vi "Library.RemoveDuplicates.vi"(8 "error in (no error)":errorcluster, 11 "Library References":refnum<vi>[](array[refnum])) -> (0 "error out":errorcluster, 3 "Library References (no duplicates)":refnum<vi>[](array[refnum]))   [LabVIEW 2011]
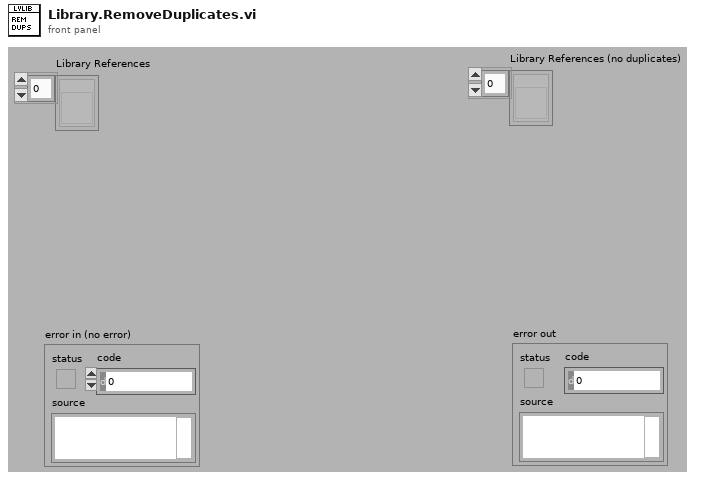
[diagram p1: front panel]
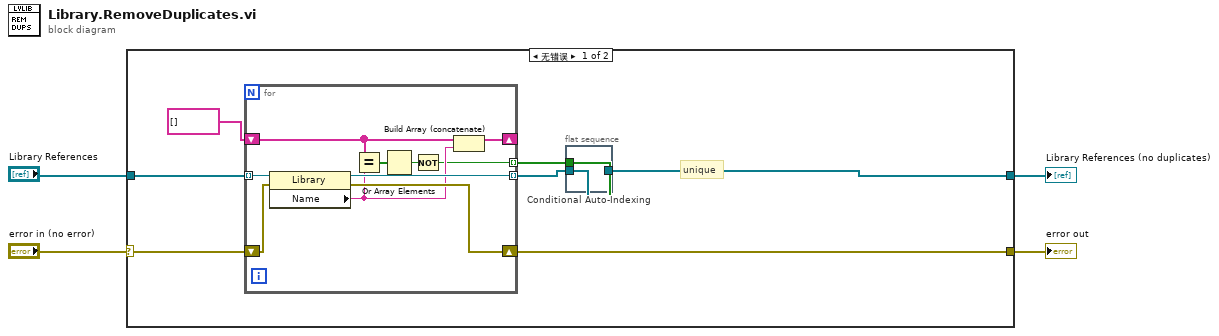
[diagram p0: block diagram]
diagram:
  n1 = case shown="无错误" "error in (no error)" {
    selector: "error in (no error)" -> [w11 w37]
    tunnel: [w7 w37] -> w4
    tunnel: "Library References" -> [w5 w36]
    tunnel: [w6 w36] -> w1
    frame No Error {
      # "unique"
      n2 = for {
        tunnel: w5 -> [w35] mode=indexing
        shift-right: [w33] -> w7
        shift-left: w11 -> [w34]
        tunnel: [w32] -> w8 mode=indexing
        shift-right: [w31] -> _
        shift-left: string[] [] -> [w29]
        tunnel: [w26] -> w9 mode=indexing
        n3 = property class="Library"(reference=w35, error in=w34) -> (reference out=w32:refnum<vi>, error out=w33:errorcluster, "Name"=w30:string)
        n4 = Equal?(x=w29, y=w30) -> (x = y?=w28:bool[])
        n5 = Or Array Elements(Boolean array=w28) -> (logical OR=w27:bool)
        n6 = Not(x=w27) -> (.not. x?=w26:bool)
        n7 = Build Array (concatenate)(w29, w30) -> (w31:string[])
      }
      n8 = flat-sequence "Conditional Auto-Indexing" {
        tunnel: w9 -> [w14]
        tunnel: w8 -> [w13]
        tunnel: [w12] -> w6
        frame #0 {
          n9 = Boolean To (0,1)(Boolean=w14) -> (0, 1=w17:i16[])
          n10 = To Unsigned Long Integer(number=w17) -> (unsigned 32bit integer=w18:u32[])
          n11 = Add Array Elements(numeric array=w18) -> (sum=w16:u32)
          n12 = for {
            N: w16 -> [_]
            tunnel: w13 -> [w21]
            tunnel: w14 -> [w25]
            shift-right: [w22] -> _
            shift-left: -1 ("start index (0)") -> [w23]
            tunnel: [w20] -> w12 mode=indexing
            # "index out that element"
            # "Find the next element to keep"
            n13 = Increment(x=w23) -> (x+1=w19:i32)
            n14 = Search 1D Array(1D array=w25, element=TRUE, start index (0)=w19) -> (index of element=w22:i32)
            n15 = Index Array(array=w21, index=w22) -> (element=w20:refnum<vi>)
          }
        }
      }
    }
    frame Error {
    }
  }
  "error out" <- w4
  "Library References (no duplicates)" <- w1
